vi "Create AO waveforms _lockin reference.vi"(9 "sampling info":cluster{"Fs":dbl, "#s":dbl}={"Fs"=1000.0, "#s"=1000.0} {"Fs" format="%.2p"}, 10 "reset signal":bool, 11 "Cluster":T1={"AO amp (V)"=[0.001, 2e-08, 0.001, 0.001, 0.001, 2e-08, 0.0, 0.0], "AO DC (V)"=[0.0, 0.0, 0.0, 0.0, 0.0, 0.0, 0.0, 0.0], "AO f (Hz)"=[13.0, 13.0, 13.0, 13.0, 13.0, 13.0, 13.0, 13.0], "AO phi (deg)"=[0.0, 0.0, 0.0, 0.0, 0.0, 0.0, 0.0, 0.0], "REF f (Hz)"=[13.0, 13.0, 13.0, 13.0, 13.0, 13.0, 13.0, 13.0], "function"=[enum."Sine Wave", enum."Sine Wave", enum."Sine Wave", enum."Sine Wave", enum."Sine Wave", enum."Sine Wave", enum."Sine Wave", enum."Sine Wave"], "REF phi (deg)"=[0.0, 0.0, 0.0, 0.0, 0.0, 0.0, 0.0, 0.0]} {"AO DC (V)" format="%#_6p"; "AO amp (V)" format="%#_6p"}) -> (0 "phase out":dbl[](array[numeric]), 1 "AO Array":waveform(dbl)[](array[waveform]), 3 "Cluster out":T1={"AO amp (V)"=[0.001, 2e-08, 0.001, 0.001, 0.001, 2e-08, 0.0, 0.0], "AO DC (V)"=[0.0, 0.0, 0.0, 0.0, 0.0, 0.0, 0.0, 0.0], "AO f (Hz)"=[13.0, 13.0, 13.0, 13.0, 13.0, 13.0, 13.0, 13.0], "AO phi (deg)"=[0.0, 0.0, 0.0, 0.0, 0.0, 0.0, 0.0, 0.0], "REF f (Hz)"=[13.0, 13.0, 13.0, 13.0, 13.0, 13.0, 13.0, 13.0], "function"=[enum."Sine Wave", enum."Sine Wave", enum."Sine Wave", enum."Sine Wave", enum."Sine Wave", enum."Sine Wave", enum."Sine Wave", enum."Sine Wave"], "REF phi (deg)"=[0.0, 0.0, 0.0, 0.0, 0.0, 0.0, 0.0, 0.0]} {"AO DC (V)" format="%#_6p"; "AO amp (V)" format="%#_6p"})   [LabVIEW 2013]
uses:
  <vilib>/measure/NI_MABase.lvlib
panel:
  out "Waveform Graph":waveform(dbl)[](graph)
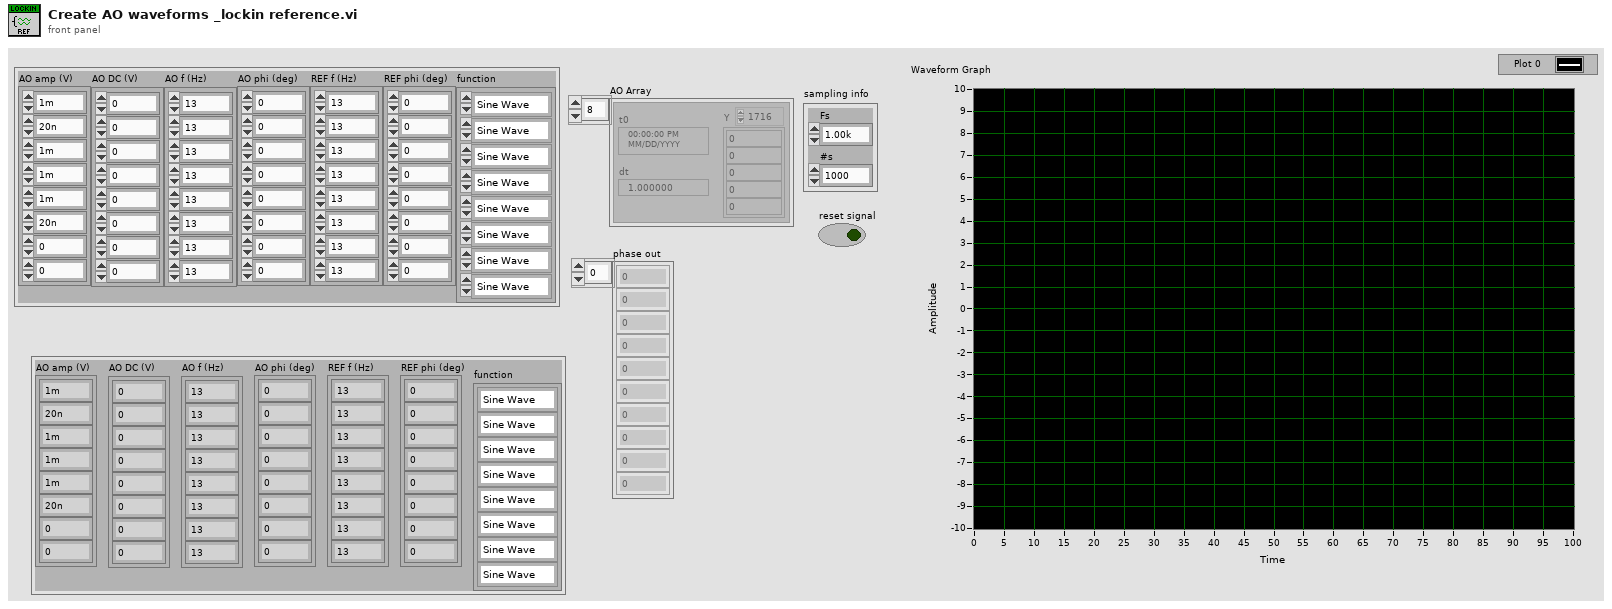
[diagram p1: front panel]
types:
  T1 = cluster{"AO amp (V)":dbl[], "AO DC (V)":dbl[], "AO f (Hz)":dbl[], "AO phi (deg)":dbl[], "REF f (Hz)":dbl[], "function":enum16{"Sine Wave", "Triangle Wave", "Square Wave", "Sawtooth Wave"}[], "REF phi (deg)":dbl[]}
  T2 = enum16{"Sine Wave", "Triangle Wave", "Square Wave", "Sawtooth Wave"}
  T3 = enum16{"Sine Wave", "Triangle Wave", "Square Wave", "Sawtooth Wave"}[]
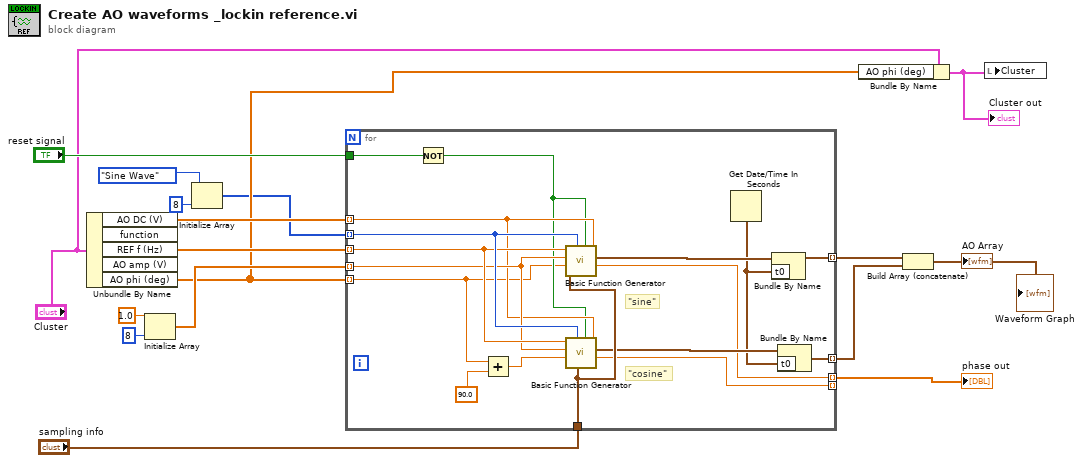
[diagram p0: block diagram]
diagram:
  n1 = Unbundle By Name("Cluster") -> ("AO DC (V)"=w17:dbl[], "REF f (Hz)"=w14:dbl[], "AO phi (deg)"=w8:dbl[])  [unwired: 2 out]
  n2 = Initialize Array(1.0 ("element"), 8 ("dimension size")) -> (w9:dbl[])
  n3 = Initialize Array(T2."Sine Wave" ("Signal Type"), 8 ("dimension size")) -> (w5:T3)
  n4 = for {
    tunnel: w5 -> [w34] mode=indexing
    tunnel: w14 -> [w33] mode=indexing
    tunnel: w9 -> [w32] mode=indexing
    tunnel: w17 -> [w31] mode=indexing
    tunnel: [w28] -> w12 mode=indexing
    tunnel: "sampling info" -> [w30]
    tunnel: [w27] -> w15 mode=indexing
    tunnel: [w22] -> w2 mode=indexing
    tunnel: [w24] -> _ mode=indexing
    tunnel: w8 -> [w18] mode=indexing
    tunnel: "reset signal" -> [w20]
    # "\"cosine\""
    # "\"sine\""
    n5 = Not(x=w20) -> (.not. x?=w19:bool)
    n6 = Add(x=w18, y=90.0) -> (x+y=w21:dbl)
    n7 = call <vilib>:"Basic Function Generator.vi"("offset"=w31, "reset signal"=w19, "sampling info"=w30, "signal type"=w34, "phase"=w18, "amplitude"=w32, "frequency"=w33) -> ("phase out"=w22:dbl, "signal out"=w29:waveform(dbl))  [unwired: 2 in, 1 out]
    n8 = call <vilib>:"Basic Function Generator.vi"("offset"=w31, "reset signal"=w19, "sampling info"=w30, "signal type"=w34, "phase"=w21, "amplitude"=w32, "frequency"=w33) -> ("phase out"=w24:dbl, "signal out"=w26:waveform(dbl))  [unwired: 2 in, 1 out]
    n9 = Get Date/Time In Seconds() -> (seconds since 1Jan1904=w25:timestamp)
    n10 = Bundle By Name(cluster=w29, "t0"=w25) -> (w28:waveform(dbl))
    n11 = Bundle By Name(cluster=w26, "t0"=w25) -> (w27:waveform(dbl))
  }
  "phase out" <- w2
  n12 = Bundle By Name(cluster="Cluster", "AO phi (deg)"=w8) -> (w3:T1)
  "Cluster out" <- w3
  n13 = Build Array (concatenate)(w12, w15) -> (→"AO Array" →"Waveform Graph":waveform(dbl)[])
  n14 = local write "Cluster"(w3) -> ()
